vi "CCE T027 SubVI02.vi"(0 "Array":u8[][](array[numeric]), 1 "UMBRAL":u8(knob) scale=0.0..255.0, 2 "INVERTIDO?":bool) -> (7 "new picture":picture, 8 "Array 2":u8[][](array[numeric]))   [LabVIEW 2020]
doc: "Ceballos Conde Emanuel Rodríguez Ramírez Miguel Ángel 4MV6 Sistemas de visión artificial 2022/1\nEste vi contiene la operacion de binarizacion para el elemento de entrada, obteninendo a la salida 1 si el valor si encuentra dentro del rango dado por el umbral superior e inferior y 0 cuando se encuentra fuera de este rango"
panel:
  # "Ceballos Conde Emanuel\n4MV6\nSistemas de visión artificial\n2022/1"
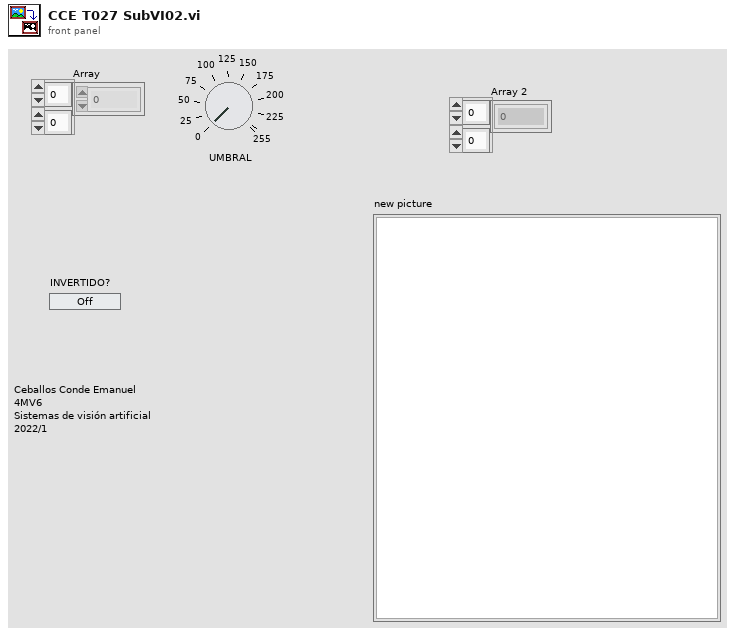
[diagram p1: front panel]
types:
  T1 = typedef "imagedata.ctl" = cluster{"image type":i32, "image depth":i32, "image":u8[], "mask":u8[], "colors":u32[], "Rectangle":cluster{"left":i16, "top":i16, "right":i16, "bottom":i16}}
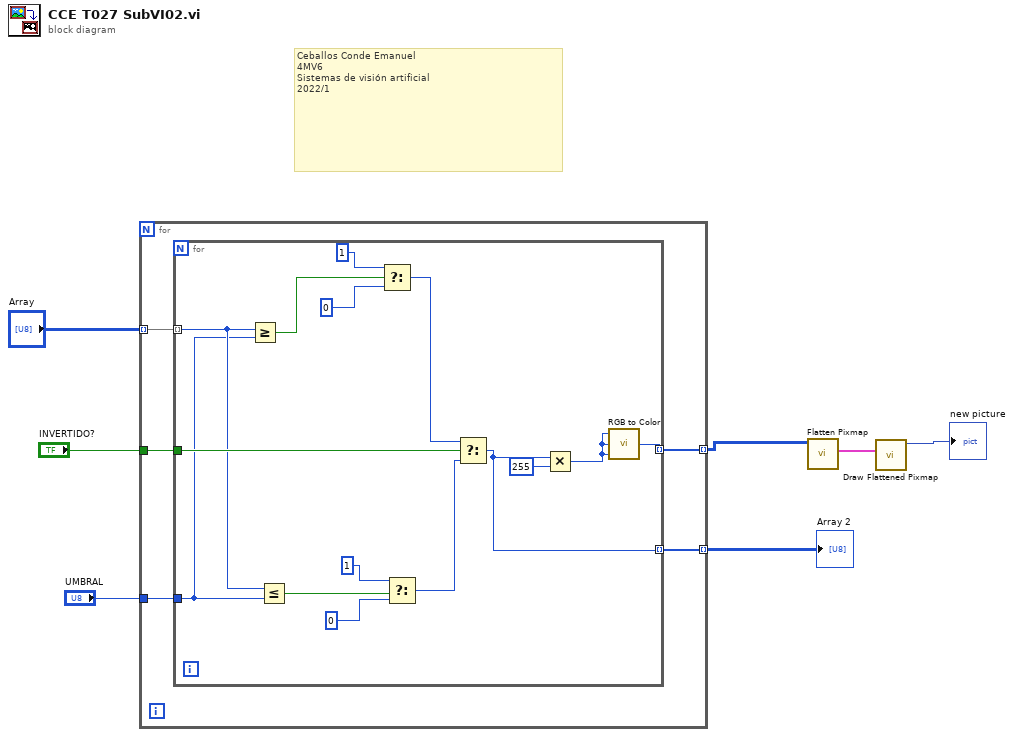
[diagram p0: block diagram]
diagram:
  # "Ceballos Conde Emanuel\n4MV6\nSistemas de visión artificial\n2022/1"
  n1 = for {
    tunnel: "INVERTIDO?" -> [w12]
    tunnel: "Array" -> [w11] mode=indexing
    tunnel: "UMBRAL" -> [w10]
    tunnel: [w9] -> w4 mode=indexing
    tunnel: [w8] -> w1 mode=indexing
    n2 = for {
      tunnel: w12 -> [w23]
      tunnel: w11 -> [w22] mode=indexing
      tunnel: w10 -> [w21]
      tunnel: [w16] -> w9 mode=indexing
      tunnel: [w15] -> w8 mode=indexing
      n3 = Greater Or Equal?(x=w22, y=w21) -> (x >= y?=w20:bool)
      n4 = Less Or Equal?(x=w22, y=w21) -> (x <= y?=w19:bool)
      n5 = Select(t=u8 1, s=w20, f=u8 0) -> (s? t:f=w17:u8)
      n6 = Select(t=u8 1, s=w19, f=u8 0) -> (s? t:f=w18:u8)
      n7 = Select(t=w17, s=w23, f=w18) -> (s? t:f=w15:u8)
      n8 = Multiply(x=w15, y=u8 255) -> (x*y=w14:u8)
      n9 = call <vilib>:"RGB to Color.vi"("B"=w14, "G"=w14, "R"=w14) -> ("Color"=w16:u32)
    }
  }
  "Array 2" <- w1
  n10 = call <vilib>:"Flatten Pixmap.vi"("24-bit pixmap"=w4) -> ("image data"=w3:T1)  [unwired: 10 in]
  n11 = call <vilib>:"Draw Flattened Pixmap.vi"("image data"=w3) -> ("new picture"=→"new picture":picture)  [unwired: 8 in]
